vi "get highest supported labview version.vi"() -> ()   [LabVIEW 2014]
uses:
  <vilib>/regexp/Match Regular Expression.xnode
panel:
  in  "files":path[](array[path])
  out "highest version file":path[](array[path])
  out "highest version":i32
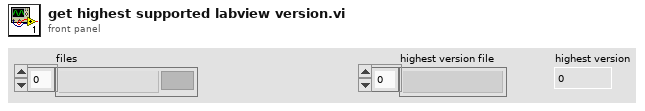
[diagram p1: front panel]
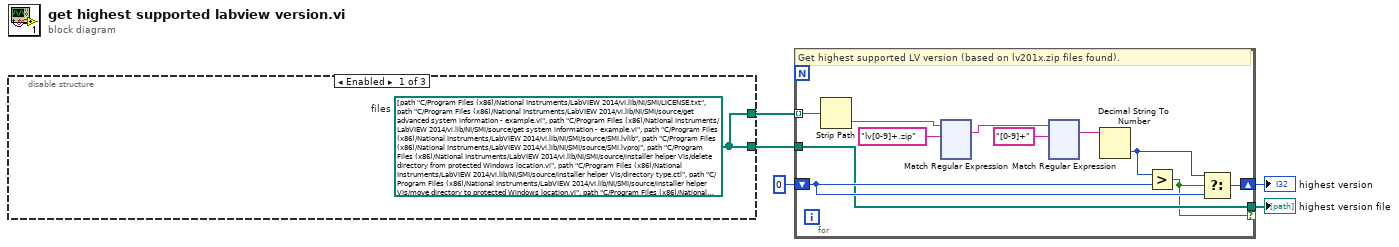
[diagram p0: block diagram]
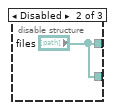
[diagram p2: hidden frame]
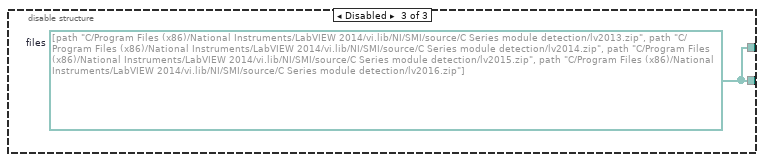
[diagram p3: hidden frame]
diagram:
  n1 = disable-structure shown="Enabled" {
    disable-tunnel: [w6 "files" w8] -> w5
    disable-tunnel: [w6 "files" w8] -> w3
    frame Enabled {
      w6 = path[] [path "C:/Program Files (x86)/National Instruments/LabVIEW 2014/vi.lib/NI/SMI/LICENSE.txt", path "C:/Program Files (x86)/National Instruments/LabVIEW 2014/vi.lib/NI/SMI/source/get advanced system information - example.vi", path "C:/Program Files (x86)/National Instruments/LabVIEW 2014/vi.lib/NI/SMI/source/get system information - example.vi", path "C:/Program Files (x86)/National Instruments/LabVIEW 2014/vi.lib/NI/SMI/source/SMI.lvlib", path "C:/Program Files (x86)/National Instruments/LabVIEW 2014/vi.lib/NI/SMI/source/SMI.lvproj", path "C:/Program Files (x86)/National Instruments/LabVIEW 2014/vi.lib/NI/SMI/source/installer helper VIs/delete directory from protected Windows location.vi", path "C:/Program Files (x86)/National Instruments/LabVIEW 2014/vi.lib/NI/SMI/source/installer helper VIs/directory type.ctl", path "C:/Program Files (x86)/National Instruments/LabVIEW 2014/vi.lib/NI/SMI/source/installer helper VIs/move directory to protected Windows location.vi", path "C:/Program Files (x86)/National Instruments/LabVIEW 2014/vi.lib/NI/SMI/source/installer helper VIs/Post-Install Custom Action.vi", path "C:/Program Files (x86)/National Instruments/LabVIEW 2014/vi.lib/NI/SMI/source/installer helper VIs/Post-Uninstall Custom Action.vi", path "C:/Program Files (x86)/National Instruments/LabVIEW 2014/vi.lib/NI/SMI/source/classes/SysCfg Device/close sys config device.vi", path "C:/Program Files (x86)/National Instruments/LabVIEW 2014/vi.lib/NI/SMI/source/classes/SysCfg Device/get network devices.vi", path "C:/Program Files (x86)/National Instruments/LabVIEW 2014/vi.lib/NI/SMI/source/classes/SysCfg Device/get sys config device information.vi", path "C:/Program Files (x86)/National Instruments/LabVIEW 2014/vi.lib/NI/SMI/source/classes/SysCfg Device/initialize sys config device.vi", path "C:/Program Files (x86)/National Instruments/LabVIEW 2014/vi.lib/NI/SMI/source/classes/SysCfg Device/read password.vi", path "C:/Program Files (x86)/National Instruments/LabVIEW 2014/vi.lib/NI/SMI/source/classes/SysCfg Device/read system session.vi", path "C:/Program Files (x86)/National Instruments/LabVIEW 2014/vi.lib/NI/SMI/source/classes/SysCfg Device/read user name.vi", path "C:/Program Files (x86)/National Instruments/LabVIEW 2014/vi.lib/NI/SMI/source/classes/SysCfg Device/real-time OS check.vi", path "C:/Program Files (x86)/National Instruments/LabVIEW 2014/vi.lib/NI/SMI/source/classes/SysCfg Device/sys config device information.ctl", path "C:/Program Files (x86)/National Instruments/LabVIEW 2014/vi.lib/NI/SMI/source/classes/SysCfg Device/SysCfg Device.lvclass", path "C:/Program Files (x86)/National Instruments/LabVIEW 2014/vi.lib/NI/SMI/source/classes/SysCfg Device/write password.vi", path "C:/Program Files (x86)/National Instruments/LabVIEW 2014/vi.lib/NI/SMI/source/classes/SysCfg Device/write sys config device object.vi", path "C:/Program Files (x86)/National Instruments/LabVIEW 2014/vi.lib/NI/SMI/source/classes/SysCfg Device/write system session.vi", path "C:/Program Files (x86)/National Instruments/LabVIEW 2014/vi.lib/NI/SMI/source/classes/SysCfg Device/write user name.vi", path "C:/Program Files (x86)/National Instruments/LabVIEW 2014/vi.lib/NI/SMI/source/classes/PXI Module/detect modules.vi", path "C:/Program Files (x86)/National Instruments/LabVIEW 2014/vi.lib/NI/SMI/source/classes/PXI Module/PXI Module.lvclass", path "C:/Program Files (x86)/National Instruments/LabVIEW 2014/vi.lib/NI/SMI/source/classes/Module/detect modules.vi", path "C:/Program Files (x86)/National Instruments/LabVIEW 2014/vi.lib/NI/SMI/source/classes/Module/get module information.vi", path "C:/Program Files (x86)/National Instruments/LabVIEW 2014/vi.lib/NI/SMI/source/classes/Module/module information.ctl", path "C:/Program Files (x86)/National Instruments/LabVIEW 2014/vi.lib/NI/SMI/source/classes/Module/Module.lvclass", path "C:/Program Files (x86)/National Instruments/LabVIEW 2014/vi.lib/NI/SMI/source/classes/Module/write module object.vi", path "C:/Program Files (x86)/National Instruments/LabVIEW 2014/vi.lib/NI/SMI/source/classes/Device/detect network devices.vi", path "C:/Program Files (x86)/National Instruments/LabVIEW 2014/vi.lib/NI/SMI/source/classes/Device/device class selection.ctl", path "C:/Program Files (x86)/National Instruments/LabVIEW 2014/vi.lib/NI/SMI/source/classes/Device/device class selection.vi", path "C:/Program Files (x86)/National Instruments/LabVIEW 2014/vi.lib/NI/SMI/source/classes/Device/device class.ctl", path "C:/Program Files (x86)/National Instruments/LabVIEW 2014/vi.lib/NI/SMI/source/classes/Device/device login credentials.ctl", path "C:/Program Files (x86)/National Instruments/LabVIEW 2014/vi.lib/NI/SMI/source/classes/Device/Device.lvclass", path "C:/Program Files (x86)/National Instruments/LabVIEW 2014/vi.lib/NI/SMI/source/classes/Device/FG action.ctl", path "C:/Program Files (x86)/National Instruments/LabVIEW 2014/vi.lib/NI/SMI/source/classes/Device/get primary NIC IP address and MAC.vi", path "C:/Program Files (x86)/National Instruments/LabVIEW 2014/vi.lib/NI/SMI/source/classes/Device/login credentials.ctl", path "C:/Program Files (x86)/National Instruments/LabVIEW 2014/vi.lib/NI/SMI/source/classes/Device/network device information.ctl", path "C:/Program Files (x86)/National Instruments/LabVIEW 2014/vi.lib/NI/SMI/source/classes/Device/read device class.vi", path "C:/Program Files (x86)/National Instruments/LabVIEW 2014/vi.lib/NI/SMI/source/classes/Device/read product ID.vi", path "C:/Program Files (x86)/National Instruments/LabVIEW 2014/vi.lib/NI/SMI/source/classes/Device/read product name.vi", path "C:/Program Files (x86)/National Instruments/LabVIEW 2014/vi.lib/NI/SMI/source/classes/Device/read serial number.vi", path "C:/Program Files (x86)/National Instruments/LabVIEW 2014/vi.lib/NI/SMI/source/classes/Device/read vendor name.vi", path "C:/Program Files (x86)/National Instruments/LabVIEW 2014/vi.lib/NI/SMI/source/classes/Device/write device class.vi", path "C:/Program Files (x86)/National Instruments/LabVIEW 2014/vi.lib/NI/SMI/source/classes/Device/write product ID.vi", path "C:/Program Files (x86)/National Instruments/LabVIEW 2014/vi.lib/NI/SMI/source/classes/Device/write product name.vi", path "C:/Program Files (x86)/National Instruments/LabVIEW 2014/vi.lib/NI/SMI/source/classes/Device/write serial number.vi", path "C:/Program Files (x86)/National Instruments/LabVIEW 2014/vi.lib/NI/SMI/source/classes/Device/write vendor name.vi", path "C:/Program Files (x86)/National Instruments/LabVIEW 2014/vi.lib/NI/SMI/source/classes/Controller/controller information.ctl", path "C:/Program Files (x86)/National Instruments/LabVIEW 2014/vi.lib/NI/SMI/source/classes/Controller/Controller.lvclass", path "C:/Program Files (x86)/National Instruments/LabVIEW 2014/vi.lib/NI/SMI/source/classes/Controller/detect chassis.vi", path "C:/Program Files (x86)/National Instruments/LabVIEW 2014/vi.lib/NI/SMI/source/classes/Controller/detect connected chassis.vi", path "C:/Program Files (x86)/National Instruments/LabVIEW 2014/vi.lib/NI/SMI/source/classes/Controller/detect controller.vi", path "C:/Program Files (x86)/National Instruments/LabVIEW 2014/vi.lib/NI/SMI/source/classes/Controller/device information.ctl", path "C:/Program Files (x86)/National Instruments/LabVIEW 2014/vi.lib/NI/SMI/source/classes/Controller/get controller information.vi", path "C:/Program Files (x86)/National Instruments/LabVIEW 2014/vi.lib/NI/SMI/source/classes/Controller/get network adapter settings.vi", path "C:/Program Files (x86)/National Instruments/LabVIEW 2014/vi.lib/NI/SMI/source/classes/Controller/network adapter settings.ctl", path "C:/Program Files (x86)/National Instruments/LabVIEW 2014/vi.lib/NI/SMI/source/classes/Controller/read device information.vi", path "C:/Program Files (x86)/National Instruments/LabVIEW 2014/vi.lib/NI/SMI/source/classes/Controller/read local chassis.vi", path "C:/Program Files (x86)/National Instruments/LabVIEW 2014/vi.lib/NI/SMI/source/classes/Controller/read primary network adapter.vi", path "C:/Program Files (x86)/National Instruments/LabVIEW 2014/vi.lib/NI/SMI/source/classes/Controller/read remote chassis.vi", path "C:/Program Files (x86)/National Instruments/LabVIEW 2014/vi.lib/NI/SMI/source/classes/Controller/read secondary network adapters.vi", path "C:/Program Files (x86)/National Instruments/LabVIEW 2014/vi.lib/NI/SMI/source/classes/Controller/read system hardware ref.vi", path "C:/Program Files (x86)/National Instruments/LabVIEW 2014/vi.lib/NI/SMI/source/classes/Controller/scan sys config device information.vi", path "C:/Program Files (x86)/National Instruments/LabVIEW 2014/vi.lib/NI/SMI/source/classes/Controller/write device information.vi", path "C:/Program Files (x86)/National Instruments/LabVIEW 2014/vi.lib/NI/SMI/source/classes/Controller/write local chassis.vi", path "C:/Program Files (x86)/National Instruments/LabVIEW 2014/vi.lib/NI/SMI/source/classes/Controller/write primary network adapter.vi", path "C:/Program Files (x86)/National Instruments/LabVIEW 2014/vi.lib/NI/SMI/source/classes/Controller/write remote chassis.vi", path "C:/Program Files (x86)/National Instruments/LabVIEW 2014/vi.lib/NI/SMI/source/classes/Controller/write secondary network adapters.vi", path "C:/Program Files (x86)/National Instruments/LabVIEW 2014/vi.lib/NI/SMI/source/classes/Controller/write system hardware ref.vi", path "C:/Program Files (x86)/National Instruments/LabVIEW 2014/vi.lib/NI/SMI/source/classes/Chassis/chassis and module information.ctl", path "C:/Program Files (x86)/National Instruments/LabVIEW 2014/vi.lib/NI/SMI/source/classes/Chassis/chassis information.ctl", path "C:/Program Files (x86)/National Instruments/LabVIEW 2014/vi.lib/NI/SMI/source/classes/Chassis/Chassis.lvclass", path "C:/Program Files (x86)/National Instruments/LabVIEW 2014/vi.lib/NI/SMI/source/classes/Chassis/detect chassis modules.vi", path "C:/Program Files (x86)/National Instruments/LabVIEW 2014/vi.lib/NI/SMI/source/classes/Chassis/get chassis information.vi", path "C:/Program Files (x86)/National Instruments/LabVIEW 2014/vi.lib/NI/SMI/source/classes/Chassis/Read modules.vi", path "C:/Program Files (x86)/National Instruments/LabVIEW 2014/vi.lib/NI/SMI/source/classes/Chassis/read number of slots.vi", path "C:/Program Files (x86)/National Instruments/LabVIEW 2014/vi.lib/NI/SMI/source/classes/Chassis/read resource name.vi", path "C:/Program Files (x86)/National Instruments/LabVIEW 2014/vi.lib/NI/SMI/source/classes/Chassis/write chassis object.vi", path "C:/Program Files (x86)/National Instruments/LabVIEW 2014/vi.lib/NI/SMI/source/classes/Chassis/Write modules.vi", path "C:/Program Files (x86)/National Instruments/LabVIEW 2014/vi.lib/NI/SMI/source/classes/Chassis/write number of slots.vi", path "C:/Program Files (x86)/National Instruments/LabVIEW 2014/vi.lib/NI/SMI/source/classes/Chassis/write resource name.vi", path "C:/Program Files (x86)/National Instruments/LabVIEW 2014/vi.lib/NI/SMI/source/classes/C Series Module/C Series Module.lvclass", path "C:/Program Files (x86)/National Instruments/LabVIEW 2014/vi.lib/NI/SMI/source/classes/C Series Module/detect modules.vi", path "C:/Program Files (x86)/National Instruments/LabVIEW 2014/vi.lib/NI/SMI/source/classes/C Series Module/module information (DAQmx).vi", path "C:/Program Files (x86)/National Instruments/LabVIEW 2014/vi.lib/NI/SMI/source/classes/C Series Module/module information (FPGA interface).vi", path "C:/Program Files (x86)/National Instruments/LabVIEW 2014/vi.lib/NI/SMI/source/classes/C Series Module/module information (scan interface).vi", path "C:/Program Files (x86)/National Instruments/LabVIEW 2014/vi.lib/NI/SMI/source/classes/C Series Module/read EEPROM addresses.vi", path "C:/Program Files (x86)/National Instruments/LabVIEW 2014/vi.lib/NI/SMI/source/classes/C Series Module/read module code (module EEPROM).vi", path "C:/Program Files (x86)/National Instruments/LabVIEW 2014/vi.lib/NI/SMI/source/classes/C Series Module/read module model (module EEPROM).vi", path "C:/Program Files (x86)/National Instruments/LabVIEW 2014/vi.lib/NI/SMI/source/classes/C Series Module/read serial number (module EEPROM).vi", path "C:/Program Files (x86)/National Instruments/LabVIEW 2014/vi.lib/NI/SMI/source/classes/C Series Module/read vendor name (module EEPROM).vi", path "C:/Program Files (x86)/National Instruments/LabVIEW 2014/vi.lib/NI/SMI/source/C Series module detection/lv2013.zip", path "C:/Program Files (x86)/National Instruments/LabVIEW 2014/vi.lib/NI/SMI/source/C Series module detection/lv2014.zip", path "C:/Program Files (x86)/National Instruments/LabVIEW 2014/vi.lib/NI/SMI/source/C Series module detection/lv2015.zip", path "C:/Program Files (x86)/National Instruments/LabVIEW 2014/vi.lib/NI/SMI/source/C Series module detection/lv2016.zip", path "C:/Program Files (x86)/National Instruments/LabVIEW 2014/vi.lib/NI/SMI/documentation/SMI Installation README.txt", path "C:/Program Files (x86)/National Instruments/LabVIEW 2014/vi.lib/NI/SMI/cdf/C Series Module Detection/2016.0.0.1/RIO_FPGA_ComboChassis.cdf", path "C:/Program Files (x86)/National Instruments/LabVIEW 2014/vi.lib/NI/SMI/cdf/C Series Module Detection/2016.0.0.1/RIO_FPGA_IntegratedChassis.cdf", path "C:/Program Files (x86)/National Instruments/LabVIEW 2014/vi.lib/NI/SMI/cdf/C Series Module Detection/2016.0.0.1/FPGABitfiles/9030_ReadEEPROM.lvbitx", path "C:/Program Files (x86)/National Instruments/LabVIEW 2014/vi.lib/NI/SMI/cdf/C Series Module Detection/2016.0.0.1/FPGABitfiles/9031_ReadEEPROM.lvbitx", path "C:/Program Files (x86)/National Instruments/LabVIEW 2014/vi.lib/NI/SMI/cdf/C Series Module Detection/2016.0.0.1/FPGABitfiles/9033_ReadEEPROM.lvbitx", path "C:/Program Files (x86)/National Instruments/LabVIEW 2014/vi.lib/NI/SMI/cdf/C Series Module Detection/2016.0.0.1/FPGABitfiles/9034_ReadEEPROM.lvbitx", path "C:/Program Files (x86)/National Instruments/LabVIEW 2014/vi.lib/NI/SMI/cdf/C Series Module Detection/2016.0.0.1/FPGABitfiles/9035_ReadEEPROM.lvbitx", path "C:/Program Files (x86)/National Instruments/LabVIEW 2014/vi.lib/NI/SMI/cdf/C Series Module Detection/2016.0.0.1/FPGABitfiles/9036_ReadEEPROM.lvbitx", path "C:/Program Files (x86)/National Instruments/LabVIEW 2014/vi.lib/NI/SMI/cdf/C Series Module Detection/2016.0.0.1/FPGABitfiles/9037_ReadEEPROM.lvbitx", path "C:/Program Files (x86)/National Instruments/LabVIEW 2014/vi.lib/NI/SMI/cdf/C Series Module Detection/2016.0.0.1/FPGABitfiles/9038_ReadEEPROM.lvbitx", path "C:/Program Files (x86)/National Instruments/LabVIEW 2014/vi.lib/NI/SMI/cdf/C Series Module Detection/2016.0.0.1/FPGABitfiles/9039_ReadEEPROM.lvbitx", path "C:/Program Files (x86)/National Instruments/LabVIEW 2014/vi.lib/NI/SMI/cdf/C Series Module Detection/2016.0.0.1/FPGABitfiles/9063_ReadEEPROM.lvbitx", path "C:/Program Files (x86)/National Instruments/LabVIEW 2014/vi.lib/NI/SMI/cdf/C Series Module Detection/2016.0.0.1/FPGABitfiles/9064_ReadEEPROM.lvbitx", path "C:/Program Files (x86)/National Instruments/LabVIEW 2014/vi.lib/NI/SMI/cdf/C Series Module Detection/2016.0.0.1/FPGABitfiles/9065_ReadEEPROM.lvbitx", path "C:/Program Files (x86)/National Instruments/LabVIEW 2014/vi.lib/NI/SMI/cdf/C Series Module Detection/2016.0.0.1/FPGABitfiles/9066_ReadEEPROM.lvbitx", path "C:/Program Files (x86)/National Instruments/LabVIEW 2014/vi.lib/NI/SMI/cdf/C Series Module Detection/2016.0.0.1/FPGABitfiles/9067_ReadEEPROM.lvbitx", path "C:/Program Files (x86)/National Instruments/LabVIEW 2014/vi.lib/NI/SMI/cdf/C Series Module Detection/2016.0.0.1/FPGABitfiles/9068_ReadEEPROM.lvbitx", path "C:/Program Files (x86)/National Instruments/LabVIEW 2014/vi.lib/NI/SMI/cdf/C Series Module Detection/2016.0.0.1/FPGABitfiles/9072_ReadEEPROM.lvbitx", path "C:/Program Files (x86)/National Instruments/LabVIEW 2014/vi.lib/NI/SMI/cdf/C Series Module Detection/2016.0.0.1/FPGABitfiles/9073_ReadEEPROM.lvbitx", path "C:/Program Files (x86)/National Instruments/LabVIEW 2014/vi.lib/NI/SMI/cdf/C Series Module Detection/2016.0.0.1/FPGABitfiles/9074_ReadEEPROM.lvbitx", path "C:/Program Files (x86)/National Instruments/LabVIEW 2014/vi.lib/NI/SMI/cdf/C Series Module Detection/2016.0.0.1/FPGABitfiles/9075_ReadEEPROM.lvbitx", path "C:/Program Files (x86)/National Instruments/LabVIEW 2014/vi.lib/NI/SMI/cdf/C Series Module Detection/2016.0.0.1/FPGABitfiles/9076_ReadEEPROM.lvbitx", path "C:/Program Files (x86)/National Instruments/LabVIEW 2014/vi.lib/NI/SMI/cdf/C Series Module Detection/2016.0.0.1/FPGABitfiles/9081_ReadEEPROM.lvbitx", path "C:/Program Files (x86)/National Instruments/LabVIEW 2014/vi.lib/NI/SMI/cdf/C Series Module Detection/2016.0.0.1/FPGABitfiles/9082_ReadEEPROM.lvbitx", path "C:/Program Files (x86)/National Instruments/LabVIEW 2014/vi.lib/NI/SMI/cdf/C Series Module Detection/2016.0.0.1/FPGABitfiles/9101_ReadEEPROM.lvbitx", path "C:/Program Files (x86)/National Instruments/LabVIEW 2014/vi.lib/NI/SMI/cdf/C Series Module Detection/2016.0.0.1/FPGABitfiles/9102_ReadEEPROM.lvbitx", path "C:/Program Files (x86)/National Instruments/LabVIEW 2014/vi.lib/NI/SMI/cdf/C Series Module Detection/2016.0.0.1/FPGABitfiles/9103_ReadEEPROM.lvbitx", path "C:/Program Files (x86)/National Instruments/LabVIEW 2014/vi.lib/NI/SMI/cdf/C Series Module Detection/2016.0.0.1/FPGABitfiles/9104_ReadEEPROM.lvbitx", path "C:/Program Files (x86)/National Instruments/LabVIEW 2014/vi.lib/NI/SMI/cdf/C Series Module Detection/2016.0.0.1/FPGABitfiles/9111_ReadEEPROM.lvbitx", path "C:/Program Files (x86)/National Instruments/LabVIEW 2014/vi.lib/NI/SMI/cdf/C Series Module Detection/2016.0.0.1/FPGABitfiles/9112_ReadEEPROM.lvbitx", path "C:/Program Files (x86)/National Instruments/LabVIEW 2014/vi.lib/NI/SMI/cdf/C Series Module Detection/2016.0.0.1/FPGABitfiles/9113_ReadEEPROM.lvbitx", path "C:/Program Files (x86)/National Instruments/LabVIEW 2014/vi.lib/NI/SMI/cdf/C Series Module Detection/2016.0.0.1/FPGABitfiles/9114_ReadEEPROM.lvbitx", path "C:/Program Files (x86)/National Instruments/LabVIEW 2014/vi.lib/NI/SMI/cdf/C Series Module Detection/2016.0.0.1/FPGABitfiles/9116_ReadEEPROM.lvbitx", path "C:/Program Files (x86)/National Instruments/LabVIEW 2014/vi.lib/NI/SMI/cdf/C Series Module Detection/2016.0.0.1/FPGABitfiles/9118_ReadEEPROM.lvbitx", path "C:/Program Files (x86)/National Instruments/LabVIEW 2014/vi.lib/NI/SMI/cdf/C Series Module Detection/2016.0.0.1/FPGABitfiles/9146_ReadEEPROM.lvbitx", path "C:/Program Files (x86)/National Instruments/LabVIEW 2014/vi.lib/NI/SMI/cdf/C Series Module Detection/2016.0.0.1/FPGABitfiles/9147_ReadEEPROM.lvbitx", path "C:/Program Files (x86)/National Instruments/LabVIEW 2014/vi.lib/NI/SMI/cdf/C Series Module Detection/2016.0.0.1/FPGABitfiles/9148_ReadEEPROM.lvbitx", path "C:/Program Files (x86)/National Instruments/LabVIEW 2014/vi.lib/NI/SMI/cdf/C Series Module Detection/2016.0.0.1/FPGABitfiles/9149_ReadEEPROM.lvbitx", path "C:/Program Files (x86)/National Instruments/LabVIEW 2014/vi.lib/NI/SMI/cdf/C Series Module Detection/2016.0.0.1/FPGABitfiles/9154_ReadEEPROM.lvbitx", path "C:/Program Files (x86)/National Instruments/LabVIEW 2014/vi.lib/NI/SMI/cdf/C Series Module Detection/2016.0.0.1/FPGABitfiles/9155_ReadEEPROM.lvbitx", path "C:/Program Files (x86)/National Instruments/LabVIEW 2014/vi.lib/NI/SMI/cdf/C Series Module Detection/2016.0.0.1/FPGABitfiles/9157_ReadEEPROM.lvbitx", path "C:/Program Files (x86)/National Instruments/LabVIEW 2014/vi.lib/NI/SMI/cdf/C Series Module Detection/2016.0.0.1/FPGABitfiles/9159_ReadEEPROM.lvbitx", path "C:/Program Files (x86)/National Instruments/LabVIEW 2014/vi.lib/NI/SMI/cdf/C Series Module Detection/2016.0.0.1/FPGABitfiles/9601_ReadEEPROM.lvbitx", path "C:/Program Files (x86)/National Instruments/LabVIEW 2014/vi.lib/NI/SMI/cdf/C Series Module Detection/2016.0.0.1/FPGABitfiles/9602_ReadEEPROM.lvbitx", path "C:/Program Files (x86)/National Instruments/LabVIEW 2014/vi.lib/NI/SMI/cdf/C Series Module Detection/2016.0.0.1/FPGABitfiles/9607_ReadEEPROM.lvbitx", path "C:/Program Files (x86)/National Instruments/LabVIEW 2014/vi.lib/NI/SMI/cdf/C Series Module Detection/2016.0.0.1/FPGABitfiles/9627_ReadEEPROM.lvbitx", path "C:/Program Files (x86)/National Instruments/LabVIEW 2014/help/System Management and Information (SMI) README.txt", path "C:/Program Files (x86)/National Instruments/LabVIEW 2014/vi.lib/addons/_functions_ni_lib_smi_1.mnu", path "C:/Program Files (x86)/National Instruments/LabVIEW 2014/vi.lib/addons/_functions_ni_lib_smi_2.mnu", path "C:/Program Files (x86)/National Instruments/LabVIEW 2014/vi.lib/addons/functions_ni_lib_smi.mnu"]  # files
    }
    frame Disabled {
    }
    frame Disabled {
      w8 = path[] [path "C:/Program Files (x86)/National Instruments/LabVIEW 2014/vi.lib/NI/SMI/source/C Series module detection/lv2013.zip", path "C:/Program Files (x86)/National Instruments/LabVIEW 2014/vi.lib/NI/SMI/source/C Series module detection/lv2014.zip", path "C:/Program Files (x86)/National Instruments/LabVIEW 2014/vi.lib/NI/SMI/source/C Series module detection/lv2015.zip", path "C:/Program Files (x86)/National Instruments/LabVIEW 2014/vi.lib/NI/SMI/source/C Series module detection/lv2016.zip"]  # files
    }
  }
  n2 = for {
    tunnel: w5 -> [w19] mode=indexing
    shift-right: [w12] -> w2
    shift-left: 0 -> [w11]
    tunnel: w3 -> [w10]
    tunnel: [w10] -> w1 if=w9
    # "Get highest supported LV version (based on lv201x.zip files found)."
    n3 = Strip Path(path=w19) -> (name=w17:string)  [unwired: 1 out]
    n4 = xnode "Match Regular Expression"("input string"=w17, "regular expression"="lv[0-9]+.zip") -> ("whole match"=w16:string)  [unwired: 4 in, 4 out]
    n5 = xnode "Match Regular Expression"("input string"=w16, "regular expression"="[0-9]+") -> ("whole match"=w14:string)  [unwired: 4 in, 4 out]
    n6 = Decimal String To Number(string=w14) -> (number=w13:i32)  [unwired: 2 in, 1 out]
    n7 = Greater?(x=w13, y=w11) -> (0:w9:bool)
    n8 = Select(t=w13, s=w9, f=w11) -> (s? t:f=w12:i32)
  }
  "highest version" <- w2
  "highest version file" <- w1
